vi "Deserialize.vi"(8 "error in (no error)":errorcluster, 10 "SerializedBoard":string) -> (0 "error out":errorcluster, 3 "Board out":refnum<class "Board.lvclass">)   [LabVIEW 2015, in "TronviewGame.lvlib" / "Board.lvclass"]
uses:
  Board.lvclass
  Board.lvclass/Board.ctl
  Serialize.vi
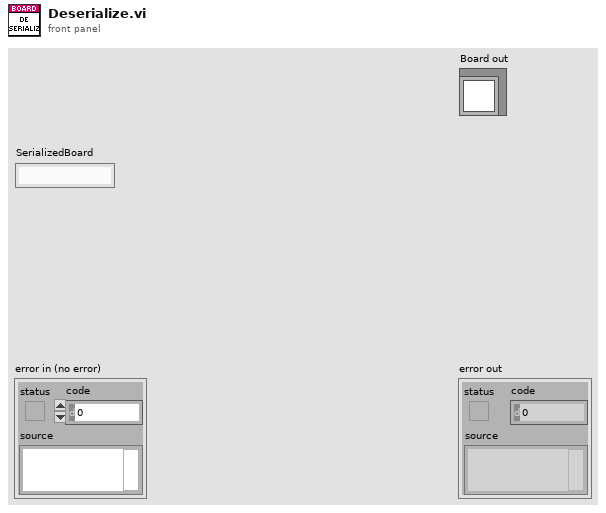
[diagram p1: front panel]
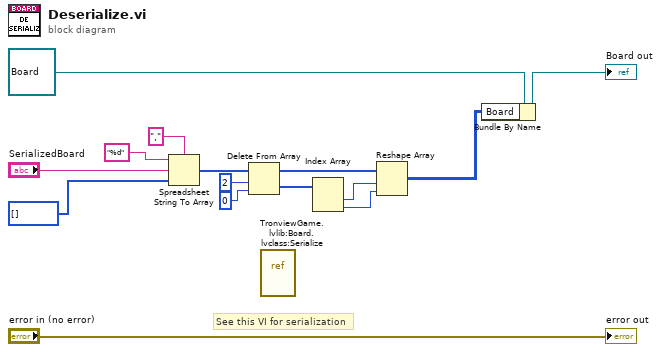
[diagram p0: block diagram]
diagram:
  # "See this VI for serialization"
  n1 = Spreadsheet String To Array(delimiter (Tab)=",", format string="%d", spreadsheet string="SerializedBoard", array type (2D Dbl)=u16[] []) -> (array=w9:u16[])
  n2 = Delete From Array(array=w9, length=2, index=0) -> (deleted portion=w5:u16[], array with subset deleted=w6:u16[])
  n3 = vi-ref "TronviewGame.lvlib:Board.lvclass:Serialize.vi"() -> ()  [unwired: 1 out]
  n4 = Index Array(array=w5) -> (element #1=w4:u16, element #2=w3:u16)  [unwired: 2 in]
  n5 = Reshape Array(w6, w4, w3) -> (w1:u16[][])
  n6 = Bundle By Name(cluster=refnum<class "Board.lvclass"> refnum ("Board in"), "Board"=w1) -> (→"Board out":refnum<class "Board.lvclass">)
  "error out" <- "error in (no error)"
